vi "Multichannel Recording0.9B.vi"() -> ()   [LabVIEW 2014]
uses:
  Enum State Typedef.ctl
  Consumer Data_ Consumer Event Com.ctl
  Data Producer States.ctl
  <vilib>/_DAQmxBase/Internals/DAQmxBase Read (Analog 2D DBL NChan NSamp).vi
  <vilib>/_DAQmxBase/Internals/DAQmxBase Create Channel (AI-Voltage-Basic).vi
  <vilib>/_DAQmxBase/Internals/DAQmxBase Timing (Sample Clock).vi
panel:
  out "Recording Progress (% )":dbl(slide) scale=0.0..1.0
  in  "Display Size":T1(ring)
  out "Total Iterations Needed":dbl
  out "Read Data":i32
  out "Data Producer State":T2=enum."Default"
  out "Data Consumer State":T3=enum."Default"
  in  "Open Button":bool
  in  "Tab Control":T4(tab)
  in  "Amplifier Channel 0":T5 {"Amplifier Model" items=["Select a Model", "AM 1700", "BMA 200"]}
  out "Channel 0 Chart":waveform(dbl)(graph)
  in  "User Data Channel 0":T6
  in  "Use Channel 0":bool caption="In Use?"
  out "Channel 1 Chart":waveform(dbl)(graph)
  in  "User Data Channel 1":T6
  in  "Amplifier Channel 1":T5 {"Amplifier Model" items=["Select a Model", "AM 1700", "BMA 200"]}
  in  "Use Channel 1":bool caption="In Use?"
  out "Channel 2 Chart":waveform(dbl)(graph)
  in  "User Data Channel 2":T6
  in  "Amplifier Channel 2":T5 {"Amplifier Model" items=["Select a Model", "AM 1700", "BMA 200"]}
  in  "Use Channel 2":bool caption="In Use?"
  out "Channel 3 Chart":waveform(dbl)(graph)
  in  "User Data Channel 3":T6
  in  "Amplifier Channel 3":T5 {"Amplifier Model" items=["Select a Model", "AM 1700", "BMA 200"]}
  in  "Use Channel 3":bool caption="In Use?"
  out "Overview Chart":waveform(dbl)[](graph)
  in  "Stop Preview":bool
  in  "OK Button":bool
  out "Event State":T7
  in  "Clear Display":bool
  in  "Preview Button":bool
  out "Iterations Recorded":i32
  in  "Recording Time (s)":dbl
  in  "Sample Rate":i64=1000
  in  "Stop Button":bool
  out "Start Time hr/min":string
  out "Date mm/dd/yy":string
  in  "Exit Button":bool
  in  "Record Button":bool
  # "MSU EFISH Lab Multi-Channel Electronic Pulse Recorder v0.9A (Beta 2)"
  # "Setup"
  # "Must set sample rate before you press start"
  # "Preview"
  # "Recording"
  # "Blue for On\nOrange for Off"
  # "DC"
  # "AC"
  # "Blue for AC and Orange for DC"
  # "Blue for On\nOrange for Off"
  # "DC"
  # "AC"
  # "Blue for AC and Orange for DC"
  # "Blue for On\nOrange for Off"
  # "DC"
  # "AC"
  # "Blue for AC and Orange for DC"
  # "Blue for On\nOrange for Off"
  # "DC"
  # "AC"
  # "Blue for AC and Orange for DC"
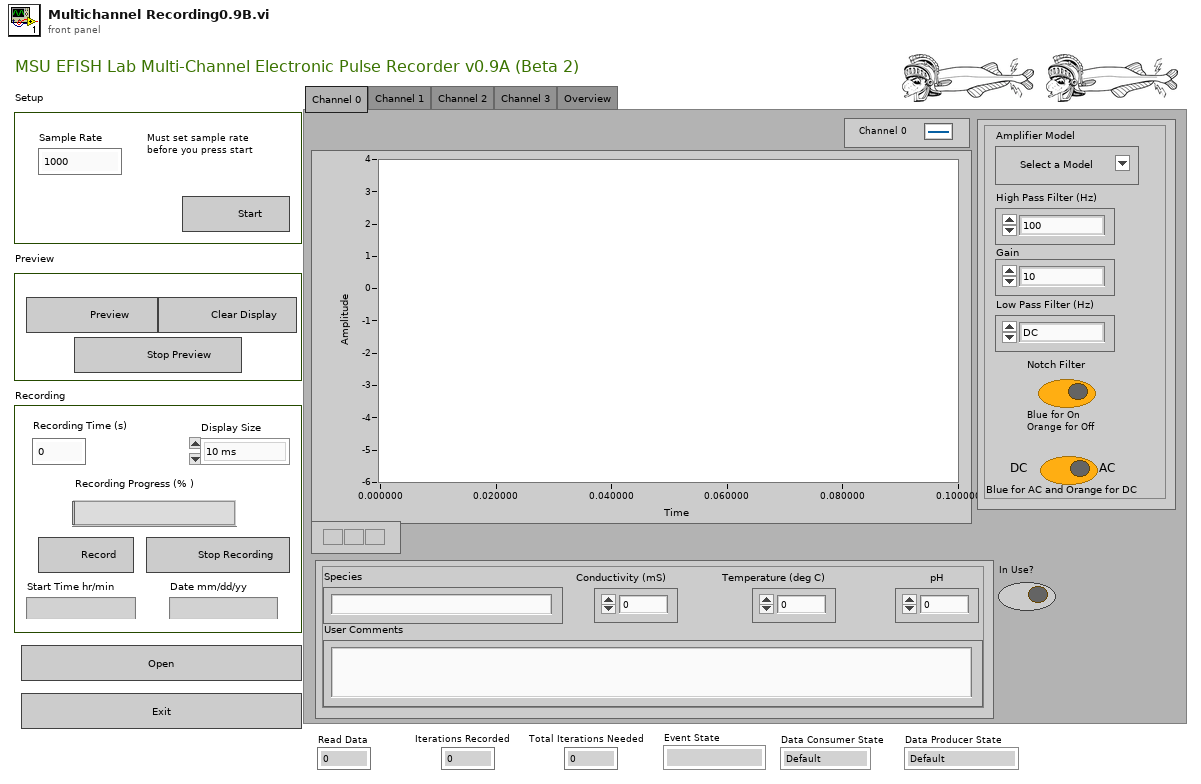
[diagram p1: front panel]
types:
  T1 = enum16{"10 ms", "100 ms", "1 Second", "10 sec", "30 sec"}
  T2 = typedef "Data Producer States.ctl" = enum16{"Read Data", "Set Sample Clock", "Default", "Exit", "Preview"}
  T3 = typedef "Consumer Data_ Consumer Event Com.ctl" = enum16{"Recording", "Create File", "Clear Memory", "Default", "End File", "Exit", "Set Sample Clock", "Preview"}
  T4 = enum32{"Channel 0", "Channel 1", "Channel 2", "Channel 3", "Overview"}
  T5 = cluster{"Low Pass Filter (Hz)":enum16{"DC", "0.1", "1", "3", "10", "30", "100", "300"}, "Gain ":enum16{"10", "20", "50", "100", "200", "500", "1000", "2k", "5k", "10k", "20k", "50k"}, "High Pass Filter (Hz)":enum16{"100", "500", "1000", "3000", "5000", "10,000", "20,000", "30,000", "50,000"}, "Notch Filter":bool, "Amplifier Model":u16, "AC/DC Switch":bool}
  T6 = cluster{"pH":dbl, "Conductivity (mS)":dbl, "Temperature (deg C)":dbl, "User Comments":string, "Species":string}
  T7 = typedef "Enum State Typedef.ctl" = enum16{"", "Open FIle", "Beginning State", "Set the Sample Clock", "Prepreview Handling", "Clear Display", "Preview Data", "Stop", "Exit", "Record", "Create File"}
  T8 = enum8{"Enabled", "Disabled", "Disabled and Grayed Out"}
  T9 = enum16{"Recording", "Create File", "Clear Memory", "Default"}
  T10 = cluster{"Refnum out":refnum<k34>, "Refnum out":refnum<k34>, "Refnum out":refnum<k34>, "Refnum out":refnum<k34>}
  T11 = cluster{"Use Channel 0":bool, "Use Channel 1":bool, "Use Channel 2":bool, "Use Channel 3":bool}
  T12 = cluster{"tdms file out":refnum<k34>, "tdms file out":refnum<k34>, "tdms file out":refnum<k34>, "tdms file out":refnum<k34>}
  T13 = cluster{"Waveform":waveform(dbl), "Waveform":waveform(dbl), "Waveform":waveform(dbl), "Waveform":waveform(dbl), waveform(dbl)[]}
  T14 = cluster{"Channel 0 Chart":refnum<vi>, "Channel 1 Chart":refnum<vi>, "Channel 2 Chart":refnum<vi>, "Channel 3 Chart":refnum<vi>, "Overview Chart":refnum<vi>}
  T15 = enum16{"Read Data", "Set Sample Clock", "Default", "Exit"}
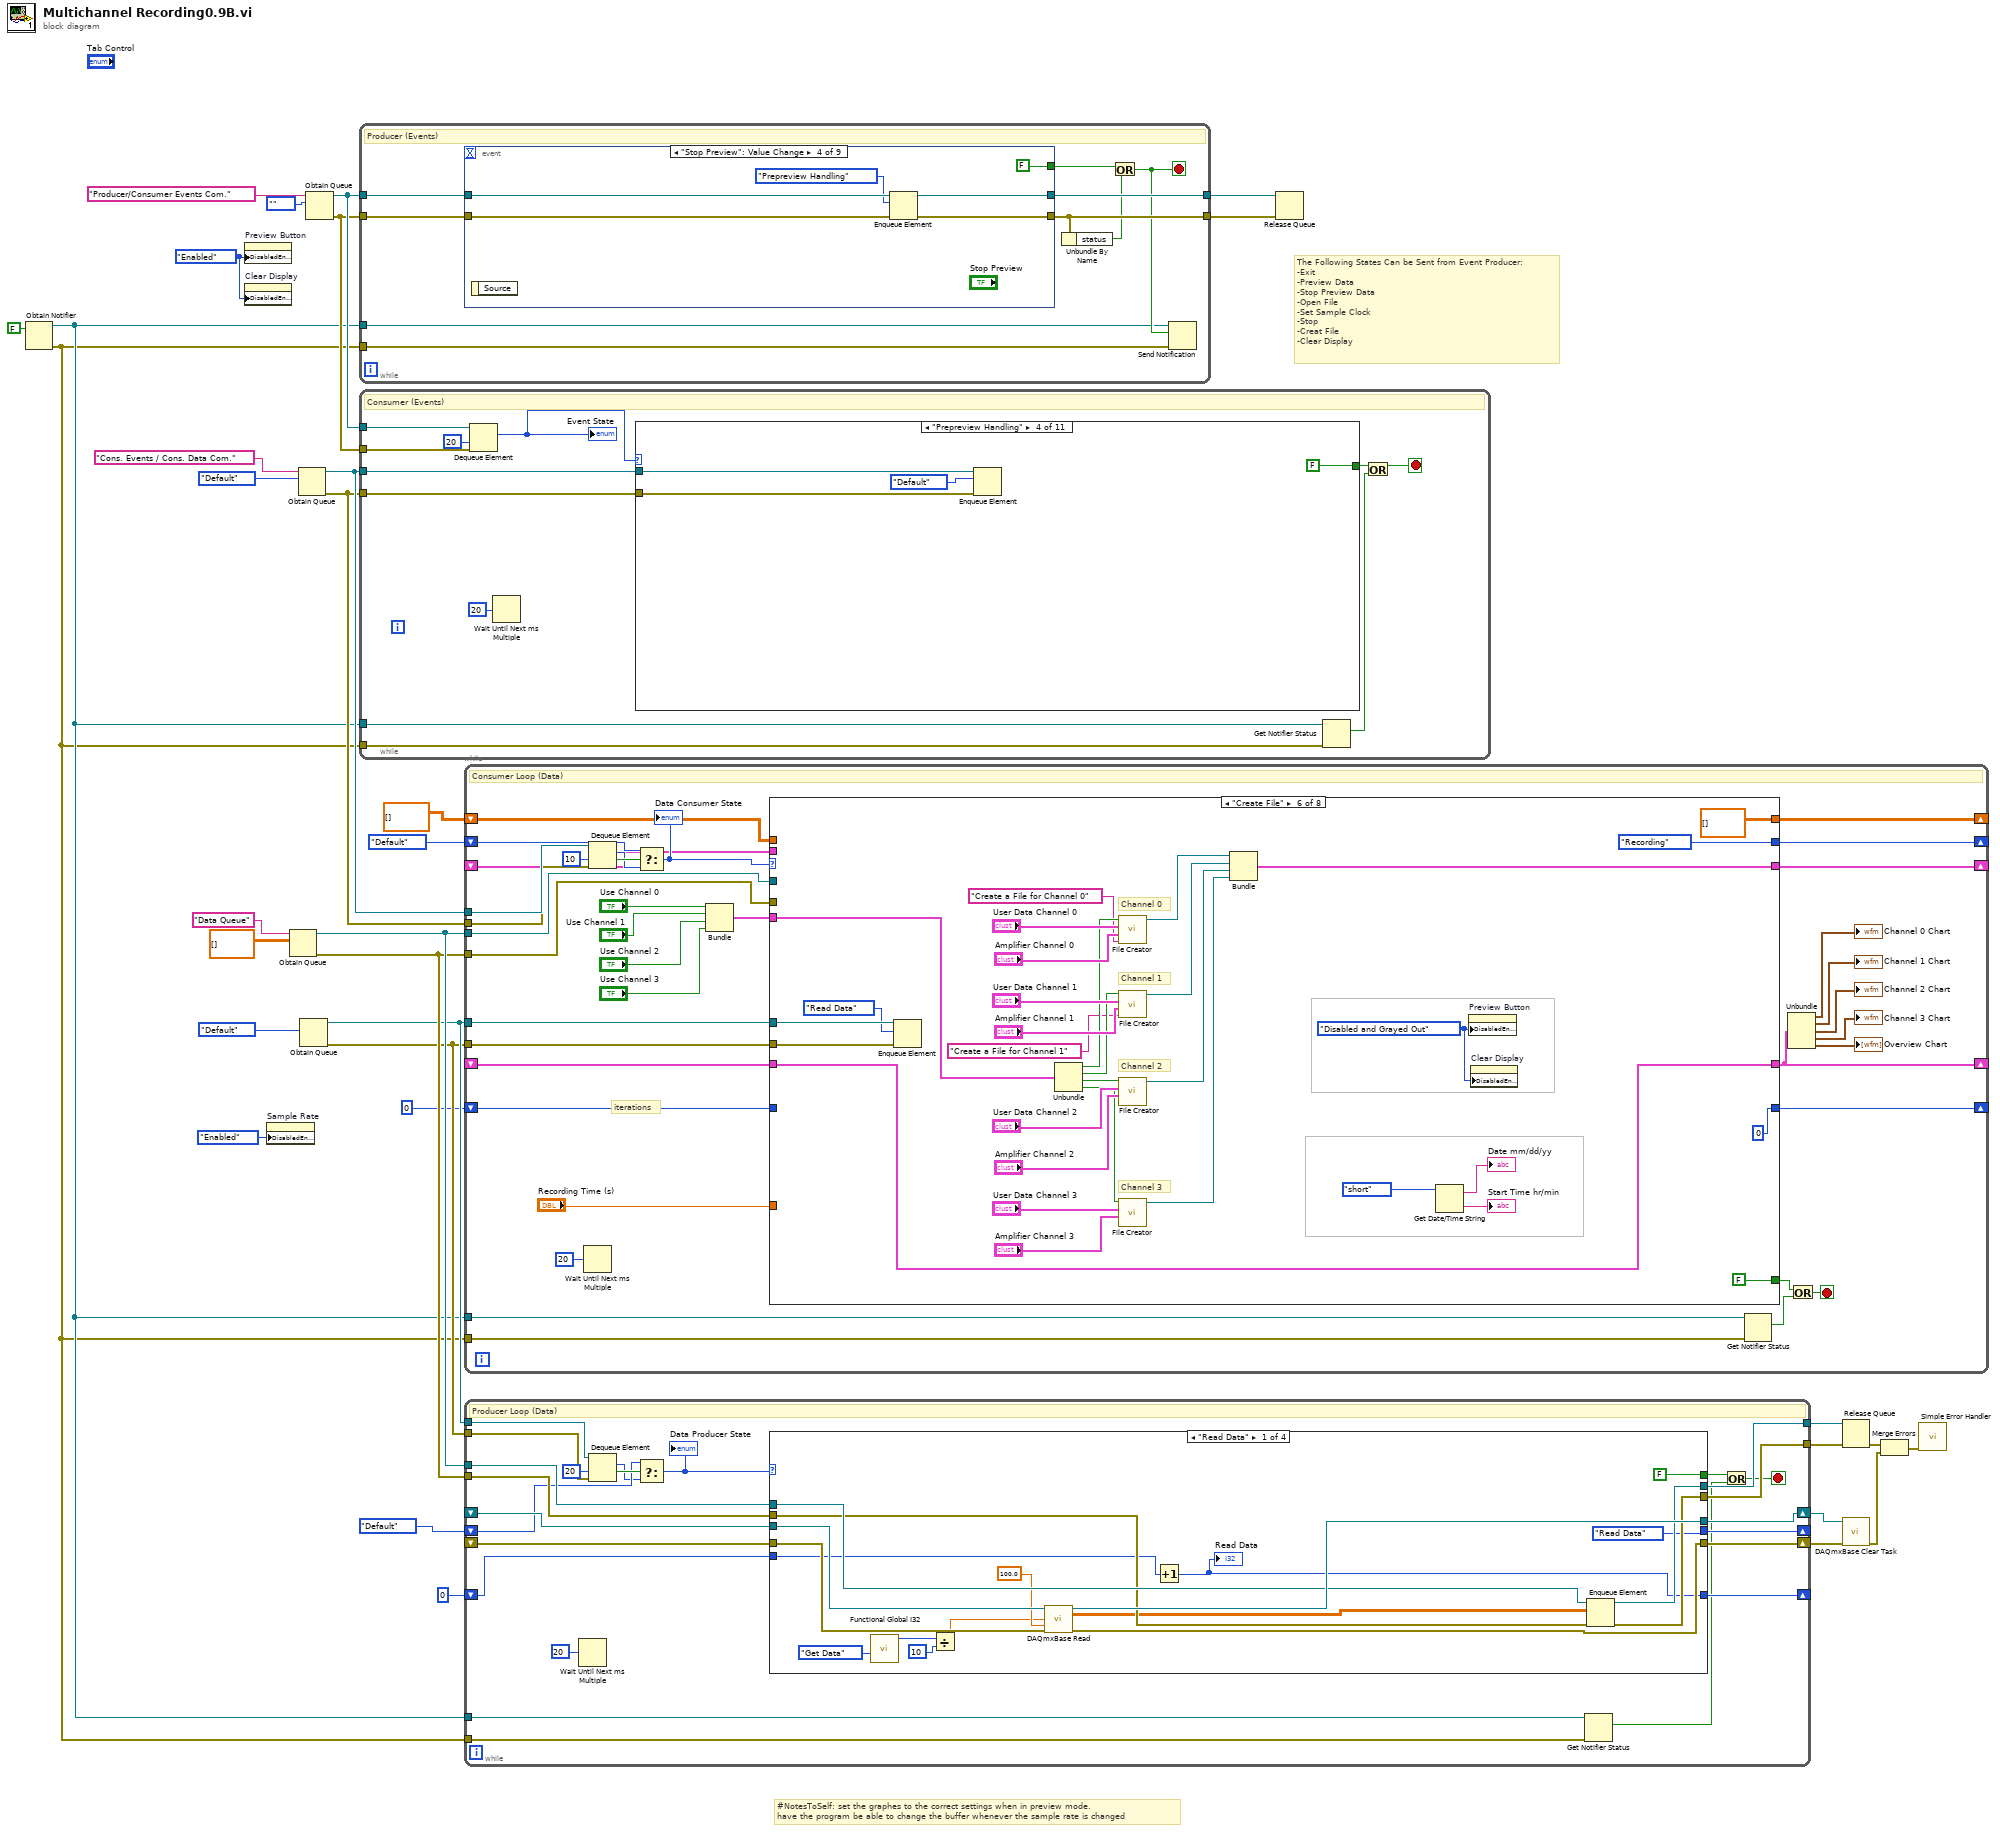
[diagram p0: block diagram]
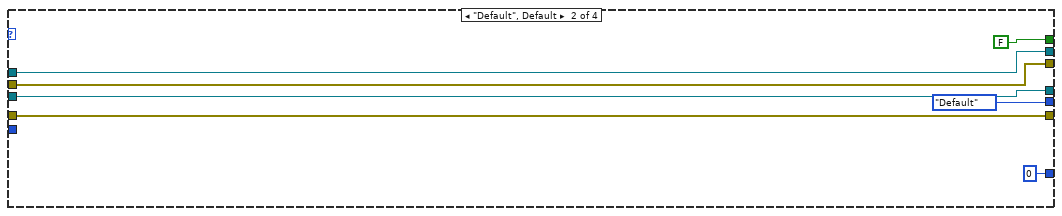
[diagram p2: hidden frame]
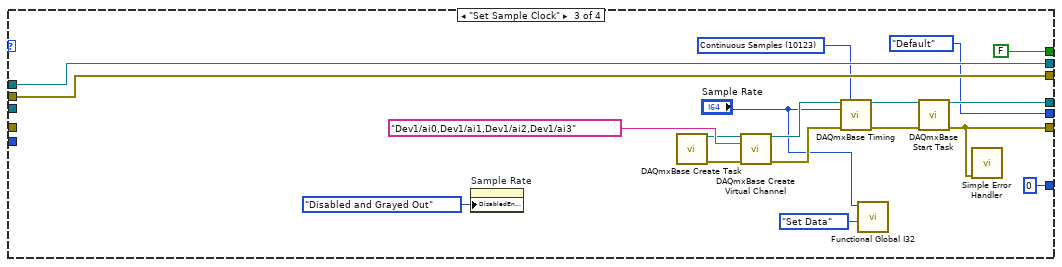
[diagram p3: hidden frame]
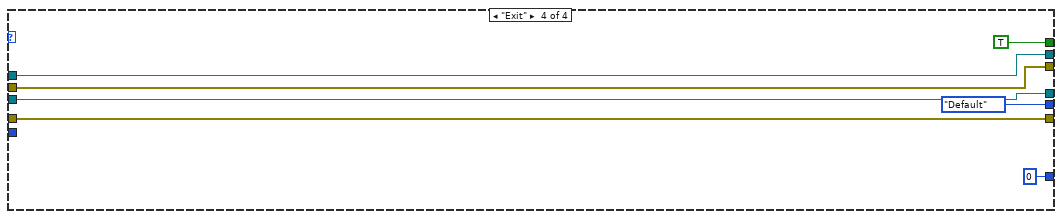
[diagram p4: hidden frame]
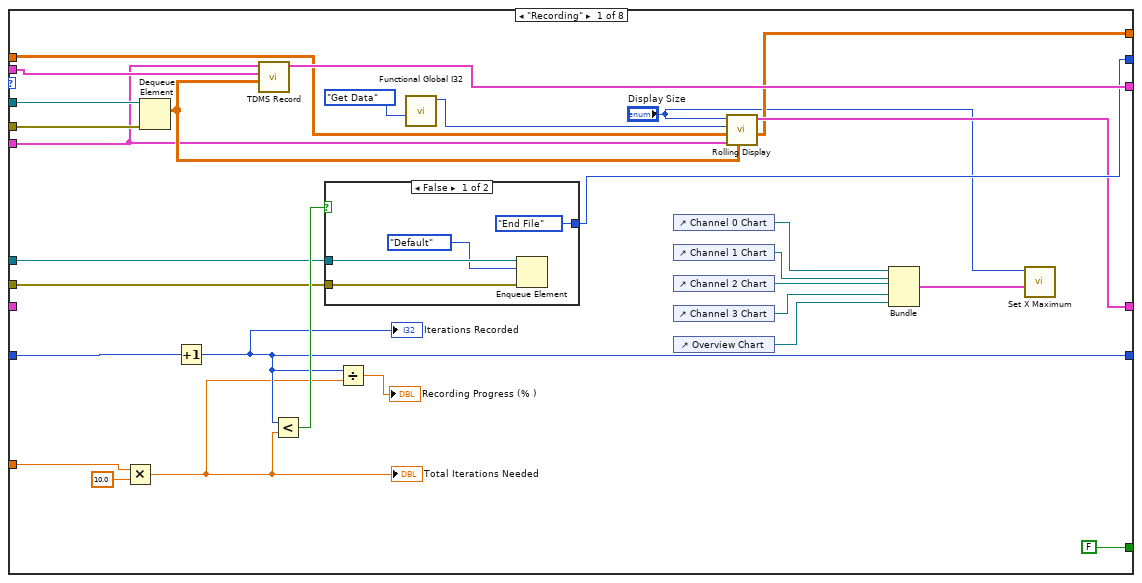
[diagram p5: hidden frame]
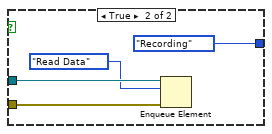
[diagram p6: hidden frame]
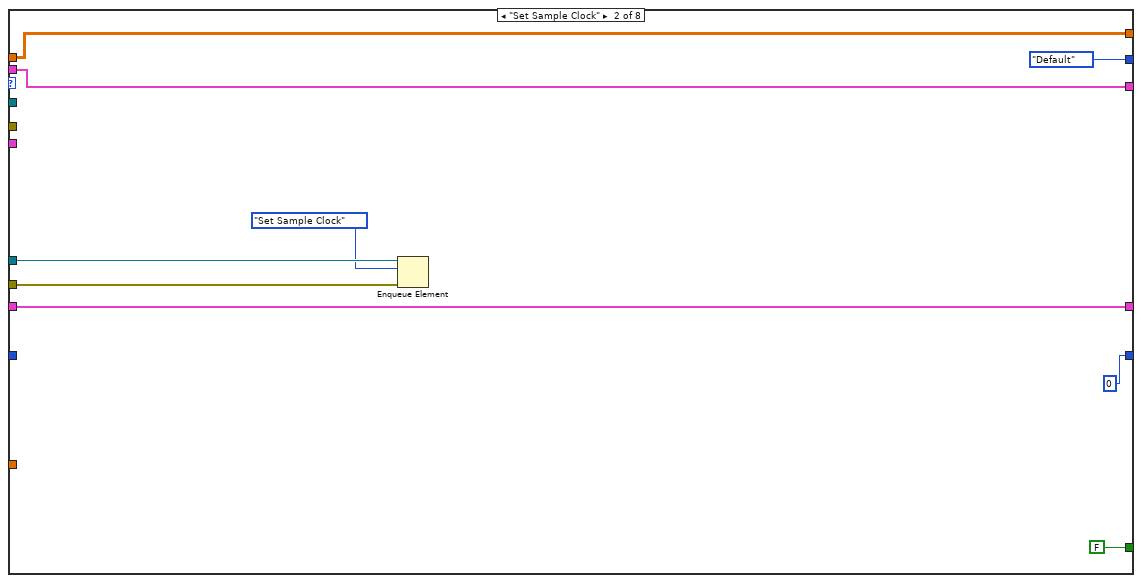
[diagram p7: hidden frame]
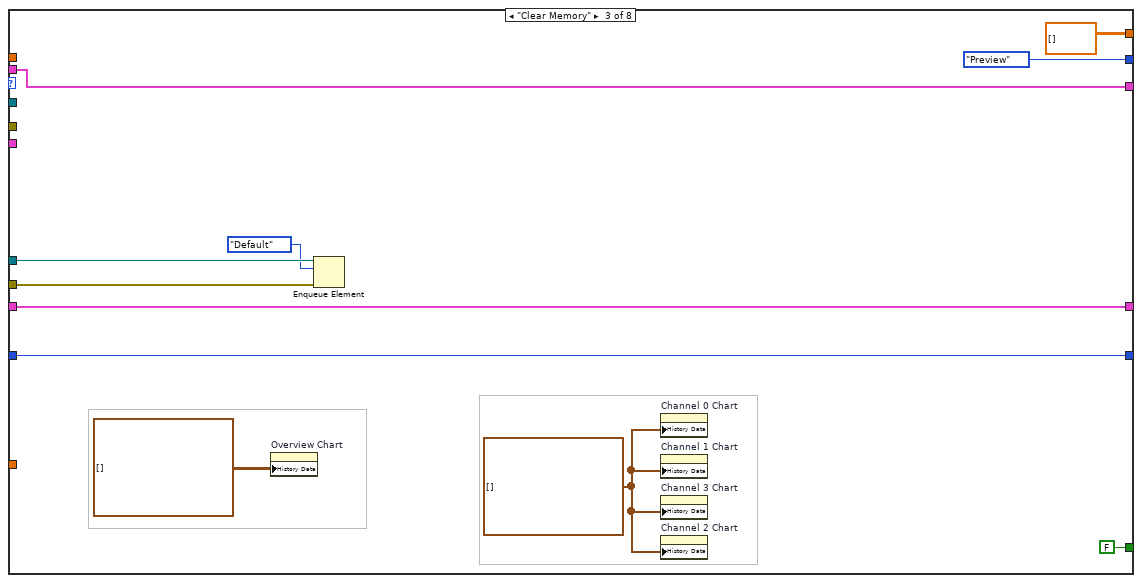
[diagram p8: hidden frame]
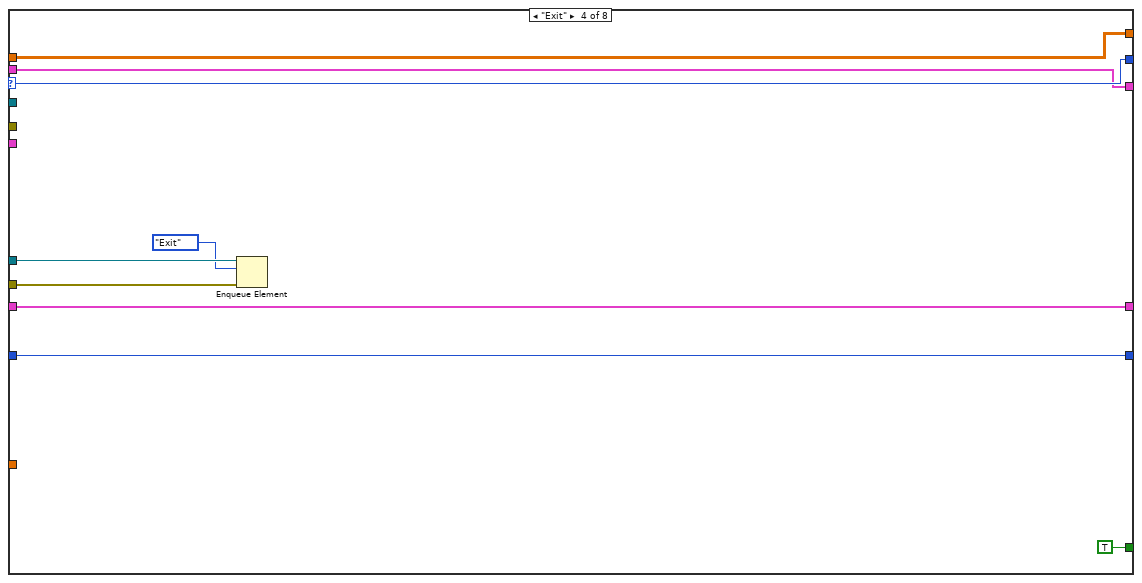
[diagram p9: hidden frame]
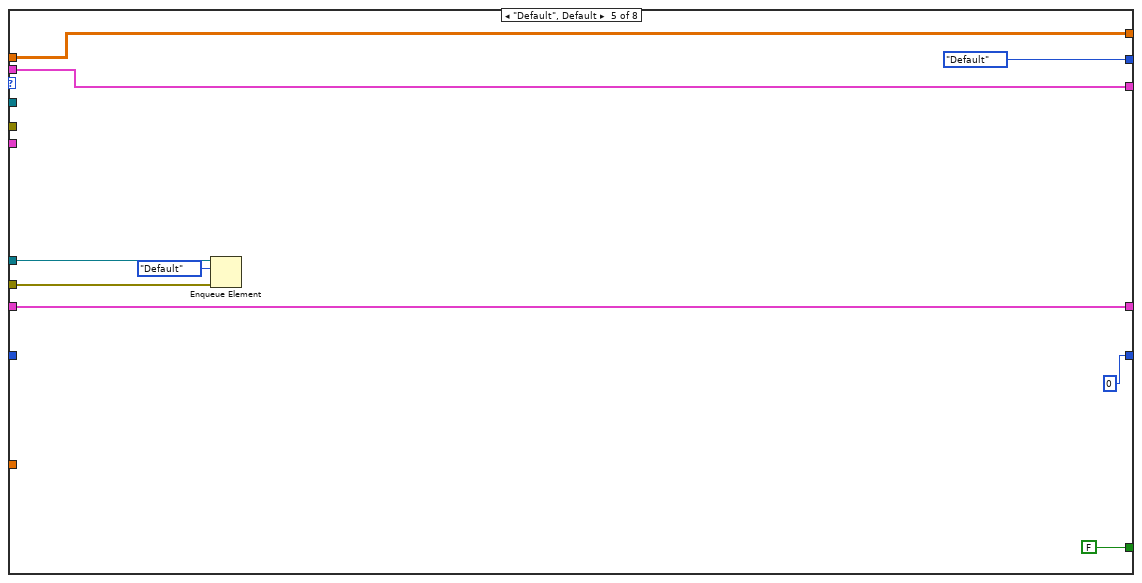
[diagram p10: hidden frame]
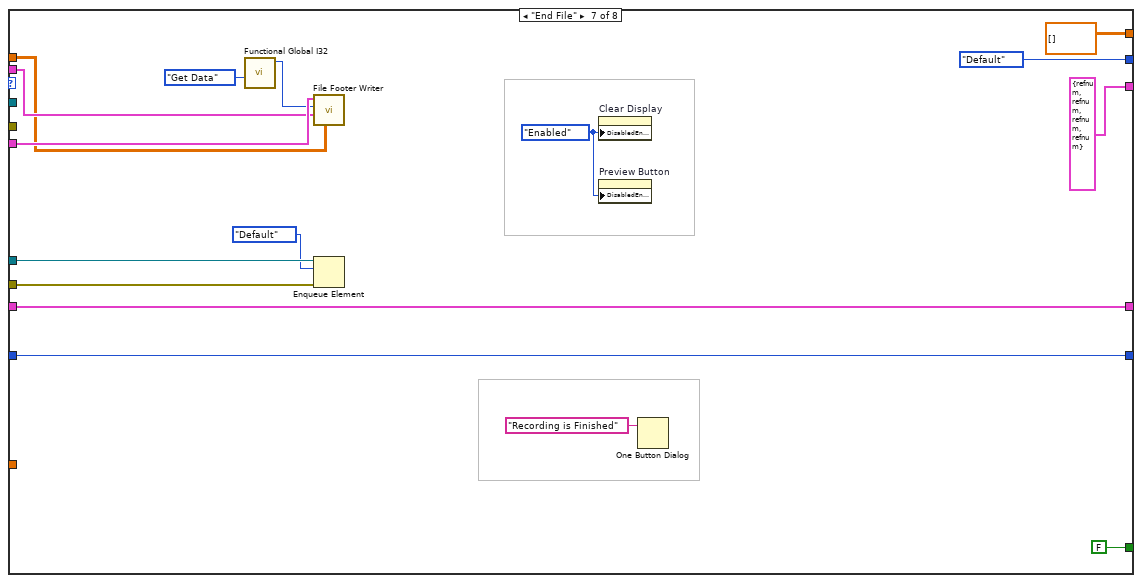
[diagram p11: hidden frame]
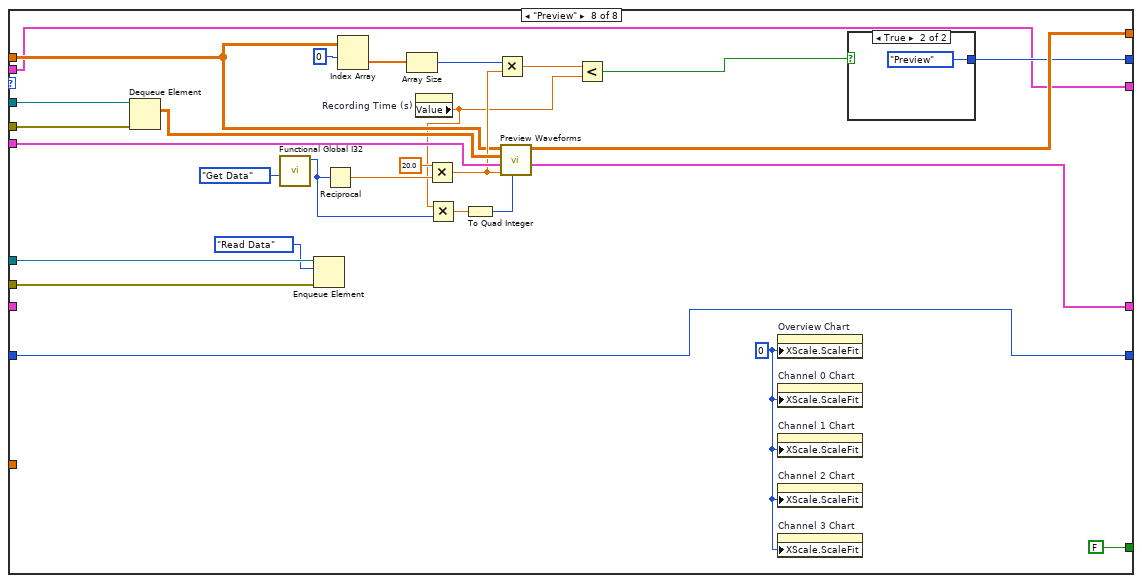
[diagram p12: hidden frame]
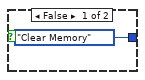
[diagram p13: hidden frame]
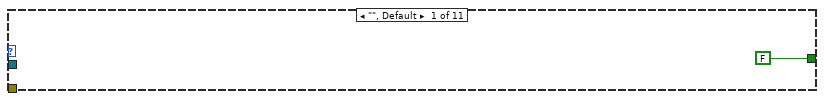
[diagram p14: hidden frame]
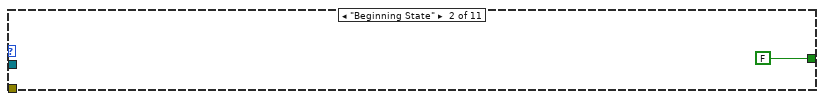
[diagram p15: hidden frame]
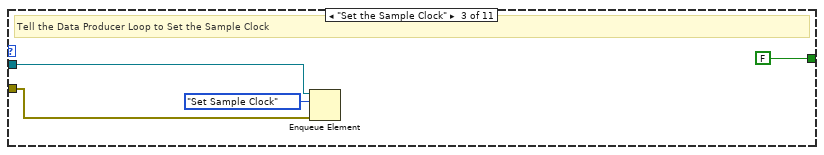
[diagram p16: hidden frame]
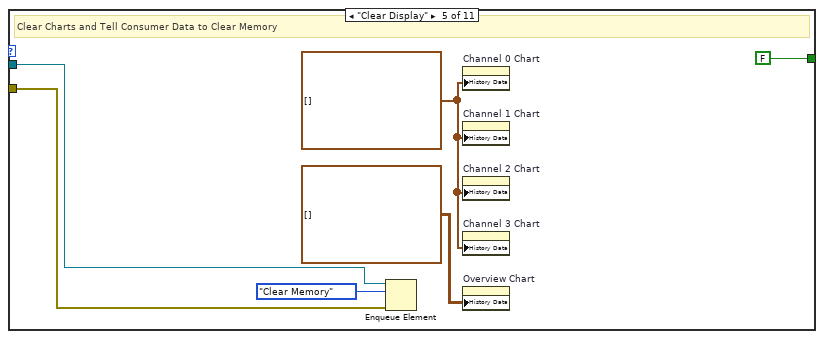
[diagram p17: hidden frame]
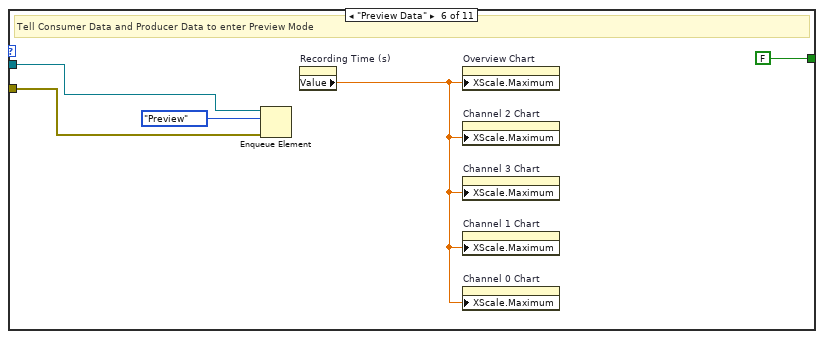
[diagram p18: hidden frame]
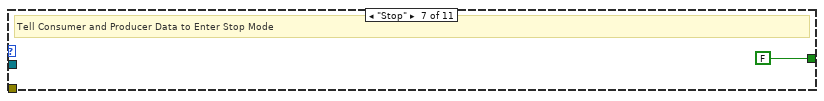
[diagram p19: hidden frame]
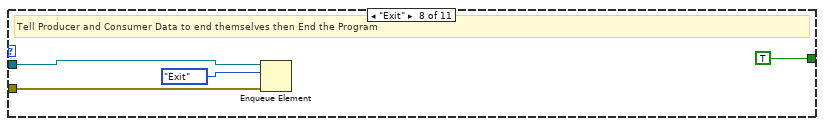
[diagram p20: hidden frame]
diagram:
  w1 = T8."Enabled" ("Disabled")
  # "#NotesToSelf: set the graphes to the correct settings when in preview mode.\nhave the program be able to change the buffer whenever the sample rate is changed"
  # "The Following States Can be Sent from Event Producer:\n-Exit\n-Preview Data\n-Stop Preview Data\n-Open File\n-Set Sample Clock\n-Stop\n-Creat File\n-Clear Display"
  n1 = Obtain Notifier(notification data type=FALSE) -> (notifier out=w3:refnum<notifier>, error out=w2:errorcluster)  [unwired: 3 in, 1 out]
  n2 = property on="Preview Button" class="Bool (strict)"("DisabledEnum"=w1) -> ()  [unwired: 2 in, 2 out]
  n3 = property on="Clear Display" class="Bool"("DisabledEnum"=w1) -> ()  [unwired: 2 in, 2 out]
  n4 = property on="Sample Rate" class="DigNum (strict)"("DisabledEnum"=T8."Enabled" ("Disabled")) -> ()  [unwired: 2 in, 2 out]
  n5 = Obtain Queue(name (unnamed)="Data Queue", element data type=dbl[][] []) -> (queue out=w29:refnum<queue>, error out=w28:errorcluster)  [unwired: 3 in, 1 out]
  n6 = Obtain Queue(name (unnamed)="Cons. Events / Cons. Data Com.", element data type=Consumer_Data__Consumer_Event_Com."Default") -> (queue out=w21:refnum<queue>, error out=w20:errorcluster)  [unwired: 3 in, 1 out]
  n7 = Obtain Queue(element data type=Data_Producer_States."Default") -> (queue out=w10:refnum<queue>, error out=w9:errorcluster)  [unwired: 4 in, 1 out]
  n8 = Obtain Queue(name (unnamed)="Producer/Consumer Events Com.", element data type=Enum_State_Typedef."" ("State")) -> (queue out=w33:refnum<queue>, error out=w32:errorcluster)  [unwired: 3 in, 1 out]
  n9 = while {
    tunnel: w33 -> [w43]
    tunnel: w32 -> [w42]
    tunnel: [w41] -> w27
    tunnel: [w40] -> w26
    tunnel: w3 -> [w36]
    tunnel: w2 -> [w35]
    stop <- w37 stop-if-true
    # "Producer (Events)"
    n10 = event shown="[3] \"Stop Preview\": Value Change" {
      selector: _ -> [_ _ _ _ _ _ _ _ _]
      dyn-events: _ -> [_ _ _ _ _ _ _ _ _]
      timeout: _ -> [_ _ _ _ _ _ _ _ _]
      tunnel: [FALSE ("Exit Button") "Exit Button" FALSE ("Exit Button") FALSE ("Exit Button") FALSE ("Exit Button") FALSE ("Exit Button") FALSE ("Exit Button") FALSE ("Exit Button") FALSE ("Exit Button")] -> w39
      tunnel: w43 -> [w45 w51 w58 w64 w70 w76 w82 w88 w94]
      tunnel: w42 -> [w44 w50 w57 w63 w69 w75 w81 w87 w93]
      tunnel: [w45 w48 w54 w60 w66 w72 w78 w84 w90] -> w41
      tunnel: [w44 w47 w53 w59 w65 w71 w77 w83 w89] -> w40
      event Timeout {
        n11 = event-data() -> ()  [unwired: 1 in, 1 out]
      }
      event "Exit Button": Value Change {
        n12 = event-data() -> ()  [unwired: 1 in, 1 out]
        n13 = Enqueue Element(queue=w51, element=Enum_State_Typedef."Exit", error in (no error)=w50) -> (queue out=w48:refnum<queue>, error out=w47:errorcluster)  [unwired: 1 in, 1 out]
      }
      event "Preview Button": Value Change {
        n14 = event-data() -> ()  [unwired: 1 in, 1 out]
        n15 = Enqueue Element(queue=w58, element=Enum_State_Typedef."Preview Data", error in (no error)=w57) -> (queue out=w54:refnum<queue>, error out=w53:errorcluster)  [unwired: 1 in, 1 out]
      }
      event "Stop Preview": Value Change {
        n16 = event-data() -> ()  [unwired: 1 in, 1 out]
        n17 = Enqueue Element(queue=w64, element=Enum_State_Typedef."Prepreview Handling", error in (no error)=w63) -> (queue out=w60:refnum<queue>, error out=w59:errorcluster)  [unwired: 1 in, 1 out]
      }
      event "Open Button": Value Change {
        n18 = event-data() -> ()  [unwired: 1 in, 1 out]
        n19 = Enqueue Element(queue=w70, element=Enum_State_Typedef."Open FIle", error in (no error)=w69) -> (queue out=w66:refnum<queue>, error out=w65:errorcluster)  [unwired: 1 in, 1 out]
      }
      event "OK Button": Value Change {
        n20 = event-data() -> ()  [unwired: 1 in, 1 out]
        n21 = Enqueue Element(queue=w76, element=Enum_State_Typedef."Set the Sample Clock", error in (no error)=w75) -> (queue out=w72:refnum<queue>, error out=w71:errorcluster)  [unwired: 1 in, 1 out]
      }
      event "Stop Button": Value Change {
        n22 = event-data() -> ()  [unwired: 1 in, 1 out]
        n23 = Enqueue Element(queue=w82, element=Enum_State_Typedef."Stop", error in (no error)=w81) -> (queue out=w78:refnum<queue>, error out=w77:errorcluster)  [unwired: 1 in, 1 out]
      }
      event "Record Button": Value Change {
        n24 = event-data() -> ()  [unwired: 1 in, 1 out]
        n25 = Enqueue Element(queue=w88, element=Enum_State_Typedef."Create File", error in (no error)=w87) -> (queue out=w84:refnum<queue>, error out=w83:errorcluster)  [unwired: 1 in, 1 out]
      }
      event "Clear Display": Value Change {
        n26 = event-data() -> ()  [unwired: 1 in, 1 out]
        n27 = Enqueue Element(queue=w94, element=Enum_State_Typedef."Clear Display", error in (no error)=w93) -> (queue out=w90:refnum<queue>, error out=w89:errorcluster)  [unwired: 1 in, 1 out]
      }
    }
    n28 = Unbundle By Name(w40) -> ("status"=w38:bool)
    n29 = Or(x=w39, y=w38) -> (x .or. y?=w37:bool)
    n30 = Send Notification(notification=w37, notifier=w36, error in (no error)=w35) -> ()  [unwired: 2 out]
  }
  n31 = while {
    tunnel: w33 -> [w106]
    tunnel: w32 -> [w105]
    tunnel: w21 -> [w104]
    tunnel: w20 -> [w103]
    tunnel: w3 -> [w98]
    tunnel: w2 -> [w97]
    stop <- w96 stop-if-true
    # "Consumer (Events)"
    n32 = Dequeue Element(queue=w106, timeout in ms (-1)=20, error in (no error)=w105) -> (element=w101:T7)  [unwired: 3 out]
    "Event State" <- w101
    n33 = Wait Until Next ms Multiple(millisecond multiple=u32 20) -> ()  [unwired: 1 out]
    n34 = case shown="\"Prepreview Handling\"" w101 {
      tunnel: w104 -> [_ _ w111 w115 w119 w125 _ w132 _ w137 _]
      tunnel: w103 -> [_ _ w110 w114 w118 w124 _ w131 _ w136 _]
      tunnel: [FALSE FALSE FALSE FALSE FALSE FALSE FALSE TRUE FALSE FALSE FALSE] -> w102
      frame "", Default {
      }
      frame "Beginning State" {
      }
      frame "Set the Sample Clock" {
        # "Tell the Data Producer Loop to Set the Sample Clock"
        n35 = Enqueue Element(queue=w111, element=Consumer_Data__Consumer_Event_Com."Set Sample Clock", error in (no error)=w110) -> ()  [unwired: 1 in, 3 out]
      }
      frame "Prepreview Handling" {
        n36 = Enqueue Element(queue=w115, element=Consumer_Data__Consumer_Event_Com."Default", error in (no error)=w114) -> ()  [unwired: 1 in, 3 out]
      }
      frame "Clear Display" {
        w121 = waveform(dbl)[] [] ("History Data")
        # "Clear Charts and Tell Consumer Data to Clear Memory"
        n37 = Enqueue Element(queue=w119, element=Consumer_Data__Consumer_Event_Com."Clear Memory", error in (no error)=w118) -> ()  [unwired: 1 in, 3 out]
        n38 = property on="Channel 0 Chart" class="WFChart (strict)"("History Data"=w121) -> ()  [unwired: 2 in, 2 out]
        n39 = property on="Channel 1 Chart" class="WFChart (strict)"("History Data"=w121) -> ()  [unwired: 2 in, 2 out]
        n40 = property on="Channel 2 Chart" class="WFChart (strict)"("History Data"=w121) -> ()  [unwired: 2 in, 2 out]
        n41 = property on="Channel 3 Chart" class="WFChart (strict)"("History Data"=w121) -> ()  [unwired: 2 in, 2 out]
        n42 = property on="Overview Chart" class="WFChart (strict)"("History Data"=waveform(dbl)[][] []) -> ()  [unwired: 2 in, 2 out]
      }
      frame "Preview Data" {
        # "Tell Consumer Data and Producer Data to enter Preview Mode"
        n43 = Enqueue Element(queue=w125, element=Consumer_Data__Consumer_Event_Com."Preview", error in (no error)=w124) -> ()  [unwired: 1 in, 3 out]
        n44 = property on="Recording Time (s)" class="DigNum (strict)"() -> ("Value"=w126:dbl)  [unwired: 2 in, 2 out]
        n45 = property on="Overview Chart" class="WFChart (strict)"("XScale.Maximum"=w126) -> ()  [unwired: 2 in, 2 out]
        n46 = property on="Channel 2 Chart" class="WFChart (strict)"("XScale.Maximum"=w126) -> ()  [unwired: 2 in, 2 out]
        n47 = property on="Channel 3 Chart" class="WFChart (strict)"("XScale.Maximum"=w126) -> ()  [unwired: 2 in, 2 out]
        n48 = property on="Channel 1 Chart" class="WFChart (strict)"("XScale.Maximum"=w126) -> ()  [unwired: 2 in, 2 out]
        n49 = property on="Channel 0 Chart" class="WFChart (strict)"("XScale.Maximum"=w126) -> ()  [unwired: 2 in, 2 out]
      }
      frame "Stop" {
        # "Tell Consumer and Producer Data to Enter Stop Mode"
      }
      frame "Exit" {
        # "Tell Producer and Consumer Data to end themselves then End the Program"
        n50 = Enqueue Element(queue=w132, element=Consumer_Data__Consumer_Event_Com."Exit", error in (no error)=w131) -> ()  [unwired: 1 in, 3 out]
      }
      frame "Record" {
        # "(I dont think that this case will exist)"
      }
      frame "Create File" {
        w134 = u8 0 ("X Scale.Scale Fit")
        # "Let Consumer Data Create File"
        n51 = Enqueue Element(queue=w137, element=Consumer_Data__Consumer_Event_Com."Create File", error in (no error)=w136) -> ()  [unwired: 1 in, 3 out]
        n52 = property on="Overview Chart" class="WFChart (strict)"("XScale.ScaleFit"=w134) -> ()  [unwired: 2 in, 2 out]
        n53 = property on="Channel 3 Chart" class="WFChart (strict)"("XScale.ScaleFit"=w134) -> ()  [unwired: 2 in, 2 out]
        n54 = property on="Channel 2 Chart" class="WFChart (strict)"("XScale.ScaleFit"=w134) -> ()  [unwired: 2 in, 2 out]
        n55 = property on="Channel 1 Chart" class="WFChart (strict)"("XScale.ScaleFit"=w134) -> ()  [unwired: 2 in, 2 out]
        n56 = property on="Channel 0 Chart" class="WFChart (strict)"("XScale.ScaleFit"=w134) -> ()  [unwired: 2 in, 2 out]
      }
      frame "Open FIle" {
        # "Tell the Data Consumer to Create the File"
        n57 = call "File Dialog"() -> ("selected path"=w139:path)  [unwired: 12 in, 3 out]
        n58 = call <vilib>:"TDMS - File Viewer.vi"("file path"=w139) -> ()  [unwired: 5 in, 2 out]
      }
    }
    n59 = Get Notifier Status(notifier=w98, error in (no error)=w97) -> (current notification=w95:bool)  [unwired: 4 out]
    n60 = Or(x=w102, y=w95) -> (x .or. y?=w96:bool)
  }
  n61 = while {
    tunnel: w29 -> [w170]
    tunnel: w28 -> [w169]
    tunnel: w21 -> [w177]
    tunnel: w20 -> [w176]
    shift-right: [w171] -> _
    shift-left: Consumer_Data__Consumer_Event_Com."Default" -> [w172]
    shift-right: [w165] -> _
    shift-left: dbl[][] [] -> [w168]
    shift-right: [w164] -> _
    shift-left: _ -> [w163]
    tunnel: w10 -> [w161]
    tunnel: w9 -> [w160]
    shift-right: [w156] -> _
    shift-left: 0 -> [w158]
    tunnel: w3 -> [w150]
    tunnel: w2 -> [w149]
    shift-right: [w142] -> _
    shift-left: _ -> [w141]
    stop <- w152 stop-if-true
    # "iterations"
    # "Consumer Loop (Data)"
    n62 = Wait Until Next ms Multiple(millisecond multiple=u32 20) -> ()  [unwired: 1 out]
    n63 = Dequeue Element(queue=w177, timeout in ms (-1)=10, error in (no error)=w176) -> (element=w174:T3, timed out?=w175:bool)  [unwired: 2 out]
    n64 = Select(t=w172, s=w175, f=w174) -> (s? t:f=w173:T3)
    "Data Consumer State" <- w173
    n65 = Bundle("Use Channel 0"="Use Channel 0", "Use Channel 1"="Use Channel 1", "Use Channel 2"="Use Channel 2", "Use Channel 3"="Use Channel 3") -> (w166:T11)  [unwired: 1 in]
    n66 = case shown="\"Create File\"" w173 {
      selector: w173 -> [_ _ _ w241 _ _ _ _]
      tunnel: [w198 Consumer_Data__Consumer_Event_Com."Default" Consumer_Data__Consumer_Event_Com."Preview" w241 T9."Default" Consumer_Data__Consumer_Event_Com."Recording" Consumer_Data__Consumer_Event_Com."Default" w314] -> w171
      tunnel: w170 -> [w205 _ _ _ _ _ _ w328]
      tunnel: w169 -> [w204 _ _ _ _ _ _ w327]
      tunnel: [FALSE FALSE FALSE TRUE FALSE FALSE FALSE FALSE] -> w151
      tunnel: w168 -> [w191 w220 _ w242 w250 _ w298 w320]
      tunnel: w166 -> [w190 _ _ _ _ w278 w300 w325]
      tunnel: [w188 w220 dbl[][] [] ("Output Decimated Data") w242 w250 dbl[][] [] ("Output Decimated Data") dbl[][] [] ("Output Data") w322] -> w165
      tunnel: [w203 w219 w231 w240 w249 w261 T10 {"Refnum out"=refnum, "Refnum out"=refnum, "Refnum out"=refnum, "Refnum out"=refnum} ("Output TDMS File Cluster") w301] -> w164
      tunnel: w163 -> [w195 w219 w231 w240 w249 _ w299 w301]
      tunnel: w161 -> [w197 w223 w228 w239 w247 w260 w293 w312]
      tunnel: w160 -> [w196 w222 w227 w238 w246 w259 w292 w311]
      tunnel: w158 -> [w202 _ w225 w236 _ _ w290 w309]
      tunnel: "Recording Time (s)" -> [w201 _ _ _ _ _ _ _]
      tunnel: [w180 0 w225 w236 0 0 w290 w309] -> w156
      tunnel: [w189 w215 w224 w235 w244 w254 w288 w306] -> w142
      tunnel: w141 -> [_ w215 w224 w235 w244 w254 w288 _]
      frame "Recording" {
        n67 = Multiply(x=w201, y=10.0) -> (x*y=w179:dbl)
        "Total Iterations Needed" <- w179
        n68 = Dequeue Element(queue=w205, error in (no error)=w204) -> (element=w192:dbl[][])  [unwired: 1 in, 3 out]
        n69 = Increment(x=w202) -> (x+1=w180:i32)
        "Iterations Recorded" <- w180
        n70 = call "TDMS Record.vi"("Data"=w192, "Input TDMS File Cluster"=w195, "In Use Cluster"=w190) -> ("Output TDMS File Cluster"=w203:T12)  [unwired: 8 in]
        n71 = Less?(x=w180, y=w179) -> (x < y?=w199:bool)
        n72 = case shown="False" w199 {
          tunnel: [Consumer_Data__Consumer_Event_Com."End File" Consumer_Data__Consumer_Event_Com."Recording"] -> w198
          tunnel: w197 -> [w209 w213]
          tunnel: w196 -> [w208 w212]
          frame False {
            n73 = Enqueue Element(queue=w209, element=Data_Producer_States."Default", error in (no error)=w208) -> ()  [unwired: 1 in, 3 out]
          }
          frame True {
            n74 = Enqueue Element(queue=w213, element=Data_Producer_States."Read Data", error in (no error)=w212) -> ()  [unwired: 1 in, 3 out]
          }
        }
        n75 = Divide(x=w180, y=w179) -> (x/y=→"Recording Progress (% )":dbl)
        n76 = call "Functional Global I32.vi"("Enum"=enum16{"Set Data", "Get Data"}."Get Data") -> ("Integer"=w193:i32)  [unwired: 10 in]
        n77 = control-ref of="Channel 0 Chart"() -> (w187:refnum<vi>)
        n78 = control-ref of="Channel 1 Chart"() -> (w186:refnum<vi>)
        n79 = control-ref of="Channel 2 Chart"() -> (w185:refnum<vi>)
        n80 = control-ref of="Channel 3 Chart"() -> (w184:refnum<vi>)
        n81 = control-ref of="Overview Chart"() -> (w183:refnum<vi>)
        n82 = call "Rolling Display.vi"("Input Data"=w192, "Channels in Use"=w190, "Old Data"=w191, "Sample Rate"=w193, "Display Size"="Display Size") -> ("Output Array Values"=w188:dbl[][], "Output Waveform Cluster"=w189:T13)  [unwired: 5 in]
        n83 = Bundle("Channel 0 Chart"=w187, "Channel 1 Chart"=w186, "Channel 2 Chart"=w185, "Channel 3 Chart"=w184, "Overview Chart"=w183) -> (w182:T14)  [unwired: 1 in]
        n84 = call "Set X Maximum.vi"("Waveform Reference Cluster"=w182, "Display Size"="Display Size") -> ()  [unwired: 10 in]
      }
      frame "Set Sample Clock" {
        n85 = Enqueue Element(queue=w223, element=Data_Producer_States."Set Sample Clock", error in (no error)=w222) -> ()  [unwired: 1 in, 3 out]
      }
      frame "Clear Memory" {
        w229 = waveform(dbl)[] [] ("History Data")
        n86 = property on="Overview Chart" class="WFChart (strict)"("History Data"=waveform(dbl)[][] []) -> ()  [unwired: 2 in, 2 out]
        n87 = Enqueue Element(queue=w228, element=Data_Producer_States."Default", error in (no error)=w227) -> ()  [unwired: 1 in, 3 out]
        n88 = property on="Channel 0 Chart" class="WFChart (strict)"("History Data"=w229) -> ()  [unwired: 2 in, 2 out]
        n89 = property on="Channel 1 Chart" class="WFChart (strict)"("History Data"=w229) -> ()  [unwired: 2 in, 2 out]
        n90 = property on="Channel 3 Chart" class="WFChart (strict)"("History Data"=w229) -> ()  [unwired: 2 in, 2 out]
        n91 = property on="Channel 2 Chart" class="WFChart (strict)"("History Data"=w229) -> ()  [unwired: 2 in, 2 out]
      }
      frame "Exit" {
        n92 = Enqueue Element(queue=w239, element=Data_Producer_States."Exit", error in (no error)=w238) -> ()  [unwired: 1 in, 3 out]
      }
      frame "Default", Default {
        n93 = Enqueue Element(queue=w247, element=Data_Producer_States."Default", error in (no error)=w246) -> ()  [unwired: 1 in, 3 out]
      }
      frame "Create File" {
        w253 = T8."Disabled and Grayed Out" ("Disabled")
        # "Channel 3"
        # "Channel 2"
        # "Channel 1"
        # "Channel 0"
        n94 = Enqueue Element(queue=w260, element=Data_Producer_States."Read Data", error in (no error)=w259) -> ()  [unwired: 1 in, 3 out]
        n95 = Unbundle(w278) -> ("Use Channel 0"=w271:bool, "Use Channel 1"=w270:bool, "Use Channel 2"=w269:bool, "Use Channel 3"=w268:bool)
        n96 = call "File Creator.vi"("prompt"="Create a File for Channel 0", "Amplifier Channel 1"="Amplifier Channel 0", "User Data Channel 1"="User Data Channel 0", "Use Channel in"=w271) -> ("Refnum out"=w267:refnum<k34>)  [unwired: 7 in]
        n97 = call "File Creator.vi"("prompt"="Create a File for Channel 1", "Amplifier Channel 1"="Amplifier Channel 1", "User Data Channel 1"="User Data Channel 1", "Use Channel in"=w270) -> ("Refnum out"=w266:refnum<k34>)  [unwired: 7 in]
        n98 = call "File Creator.vi"("Amplifier Channel 1"="Amplifier Channel 2", "User Data Channel 1"="User Data Channel 2", "Use Channel in"=w269) -> ("Refnum out"=w265:refnum<k34>)  [unwired: 8 in]
        n99 = call "File Creator.vi"("Amplifier Channel 1"="Amplifier Channel 3", "User Data Channel 1"="User Data Channel 3", "Use Channel in"=w268) -> ("Refnum out"=w264:refnum<k34>)  [unwired: 8 in]
        n100 = Bundle("Refnum out"=w267, "Refnum out"=w266, "Refnum out"=w265, "Refnum out"=w264) -> (w261:T10)  [unwired: 1 in]
        n101 = Get Date/Time String(date format (0)=enum16{"short", "long", "abbreviated"}."short") -> (date string=→"Date mm/dd/yy":string, time string=→"Start Time hr/min":string)  [unwired: 2 in]
        n102 = property on="Preview Button" class="Bool (strict)"("DisabledEnum"=w253) -> ()  [unwired: 2 in, 2 out]
        n103 = property on="Clear Display" class="Bool"("DisabledEnum"=w253) -> ()  [unwired: 2 in, 2 out]
      }
      frame "End File" {
        w287 = T8."Enabled" ("Disabled")
        n104 = call "Functional Global I32.vi"("Enum"=enum16{"Set Data", "Get Data"}."Get Data") -> ("Integer"=w285:i32)  [unwired: 10 in]
        n105 = call "File Footer Writer.vi"("Old Data"=w298, "TDMS File Cluster"=w299, "Sample Rate"=w285, "In Use Cluster"=w300) -> ()  [unwired: 8 in]
        n106 = Enqueue Element(queue=w293, element=Data_Producer_States."Default", error in (no error)=w292) -> ()  [unwired: 1 in, 3 out]
        n107 = property on="Clear Display" class="Bool"("DisabledEnum"=w287) -> ()  [unwired: 2 in, 2 out]
        n108 = property on="Preview Button" class="Bool (strict)"("DisabledEnum"=w287) -> ()  [unwired: 2 in, 2 out]
        n109 = One Button Dialog(message="Recording is Finished") -> ()  [unwired: 1 in, 1 out]
      }
      frame "Preview" {
        w307 = u8 0 ("X Scale.Scale Fit")
        n110 = Dequeue Element(queue=w328, error in (no error)=w327) -> (element=w326:dbl[][])  [unwired: 1 in, 3 out]
        n111 = call "Functional Global I32.vi"("Enum"=enum16{"Set Data", "Get Data"}."Get Data") -> ("Integer"=w305:i32)  [unwired: 10 in]
        n112 = Enqueue Element(queue=w312, element=Data_Producer_States."Read Data", error in (no error)=w311) -> ()  [unwired: 1 in, 3 out]
        n113 = Reciprocal(x=w305) -> (1/x=w324:dbl)
        n114 = Index Array(array=w320, index (row)=0) -> (element=w318:dbl[])  [unwired: 1 in]
        n115 = Array Size(array=w318) -> (size(s)=w317:i32)
        n116 = property on="Recording Time (s)" class="DigNum (strict)"() -> ("Value"=w304:dbl)  [unwired: 2 in, 2 out]
        n117 = Multiply(x=20.0, y=w324) -> (x*y=w321:dbl)
        n118 = Multiply(x=w304, y=w305) -> (x*y=w303:dbl)
        n119 = To Quad Integer(1:w303) -> (0:w302:i64)
        n120 = Multiply(x=w317, y=w321) -> (x*y=w316:dbl)
        n121 = call "Preview Waveforms.vi"("Max Size"=w302, "Change in Time"=w321, "In Use Cluster"=w325, "Input Read Data"=w326, "Input Decimated Data"=w320) -> ("Output Waveform Cluster"=w306:T13, "Output Data"=w322:dbl[][])  [unwired: 5 in]
        n122 = Less?(x=w316, y=w304) -> (x < y?=w315:bool)
        n123 = property on="Overview Chart" class="WFChart (strict)"("XScale.ScaleFit"=w307) -> ()  [unwired: 2 in, 2 out]
        n124 = property on="Channel 0 Chart" class="WFChart (strict)"("XScale.ScaleFit"=w307) -> ()  [unwired: 2 in, 2 out]
        n125 = property on="Channel 1 Chart" class="WFChart (strict)"("XScale.ScaleFit"=w307) -> ()  [unwired: 2 in, 2 out]
        n126 = property on="Channel 2 Chart" class="WFChart (strict)"("XScale.ScaleFit"=w307) -> ()  [unwired: 2 in, 2 out]
        n127 = property on="Channel 3 Chart" class="WFChart (strict)"("XScale.ScaleFit"=w307) -> ()  [unwired: 2 in, 2 out]
        n128 = case shown="True" w315 {
          tunnel: [Consumer_Data__Consumer_Event_Com."Clear Memory" Consumer_Data__Consumer_Event_Com."Preview"] -> w314
          frame False {
          }
          frame True {
          }
        }
      }
    }
    n129 = Get Notifier Status(notifier=w150, error in (no error)=w149) -> (current notification=w148:bool)  [unwired: 4 out]
    n130 = Unbundle(w142) -> ("Waveform"=→"Channel 0 Chart":waveform(dbl), "Waveform"=→"Channel 1 Chart":waveform(dbl), "Waveform"=→"Channel 2 Chart":waveform(dbl), "Waveform"=→"Channel 3 Chart":waveform(dbl), →"Overview Chart":waveform(dbl)[])
    n131 = Or(x=w151, y=w148) -> (x .or. y?=w152:bool)
  }
  n132 = while {
    tunnel: w29 -> [w354]
    tunnel: w28 -> [w351]
    tunnel: [w353] -> w25
    tunnel: [w352] -> w24
    shift-right: [w339] -> _
    shift-left: Data_Producer_States."Default" -> [w332]
    shift-right: [w350] -> w18
    shift-left: _ -> [w348]
    shift-right: [w349] -> w17
    shift-left: _ -> [w347]
    tunnel: w10 -> [w344]
    tunnel: w9 -> [w343]
    shift-right: [w337] -> _
    shift-left: 0 -> [w338]
    tunnel: w3 -> [w334]
    tunnel: w2 -> [w333]
    stop <- w336 stop-if-true
    # "Producer Loop (Data)"
    n133 = Wait Until Next ms Multiple(millisecond multiple=u32 20) -> ()  [unwired: 1 out]
    n134 = Dequeue Element(queue=w344, timeout in ms (-1)=20, error in (no error)=w343) -> (element=w331:T2, timed out?=w342:bool)  [unwired: 2 out]
    n135 = Select(t=w332, s=w342, f=w331) -> (s? t:f=w341:T2)
    "Data Producer State" <- w341
    n136 = case shown="\"Read Data\"" w341 {
      tunnel: w354 -> [w368 w379 w389 w400]
      tunnel: [w366 w379 w389 w400] -> w353
      tunnel: [w365 w378 w388 w401] -> w352
      tunnel: w351 -> [w367 w378 w388 w401]
      tunnel: [w370 w377 w390 w402] -> w350
      tunnel: [w369 w376 w380 w403] -> w349
      tunnel: w348 -> [w372 w377 _ w402]
      tunnel: w347 -> [w371 w376 _ w403]
      tunnel: [FALSE FALSE FALSE TRUE] -> w345
      tunnel: [Data_Producer_States."Read Data" Data_Producer_States."Default" T15."Default" Data_Producer_States."Default"] -> w339
      tunnel: w338 -> [w361 _ _ _]
      tunnel: [w360 0 0 0] -> w337
      frame "Read Data" {
        n137 = call "Functional Global I32.vi"("Enum"=enum16{"Set Data", "Get Data"}."Get Data") -> ("Integer"=w357:i32)  [unwired: 10 in]
        n138 = Divide(x=w357, y=10) -> (x/y=w356:dbl)
        n139 = call-poly <vilib>:"DAQmxBase Read.vi"("task/channels in"=w372, "number of samples per channel"=w356, "timeout"=100.0, "error in"=w371) -> ("task out"=w370:refnum<k21>, "data"=w355:dbl[][], "error out"=w369:errorcluster)  [unwired: 9 in]
        n140 = Increment(x=w361) -> (x+1=w360:i32)
        "Read Data" <- w360
        n141 = Enqueue Element(queue=w368, element=w355, error in (no error)=w367) -> (queue out=w366:refnum<queue>, error out=w365:errorcluster)  [unwired: 1 in, 1 out]
      }
      frame "Default", Default {
      }
      frame "Set Sample Clock" {
        w381 = 10123 items=["Finite Samples"=10178, "Continuous Samples"=10123, "Hardware Timed Single Point"=12522] ("sample mode")
        n142 = property on="Sample Rate" class="DigNum (strict)"("DisabledEnum"=T8."Disabled and Grayed Out" ("Disabled")) -> ()  [unwired: 2 in, 2 out]
        n143 = call <vilib>:"DAQmxBase Create Task.vi"() -> ("task out"=w396:refnum<k21>, "error out"=w395:errorcluster)  [unwired: 14 in]
        n144 = call-poly <vilib>:"DAQmxBase Create Virtual Channel.vi"("task in"=w396, "physical channels"=tag "Dev1/ai0,Dev1/ai1,Dev1/ai2,Dev1/ai3", "error in"=w395) -> ("task out"=w393:refnum<k21>, "error out"=w394:errorcluster)  [unwired: 11 in]
        n145 = call-poly <vilib>:"DAQmxBase Timing.vi"("task/channels in"=w393, "sample mode"=w381, "rate"="Sample Rate", "error in"=w394) -> ("task out"=w392:refnum<k21>, "error out"=w391:errorcluster)  [unwired: 10 in]
        n146 = call "Functional Global I32.vi"("Enum"=enum16{"Set Data", "Get Data"}."Set Data", "Integer In"="Sample Rate") -> ()  [unwired: 9 in, 1 out]
        n147 = call <vilib>:"DAQmxBase Start Task.vi"("task/channels in"=w392, "error in"=w391) -> ("task out"=w390:refnum<k21>, "error out"=w380:errorcluster)  [unwired: 12 in]
        n148 = call <vilib>:"Simple Error Handler.vi"("error in (no error)"=w380) -> ()  [unwired: 4 in, 5 out]
      }
      frame "Exit" {
      }
    }
    n149 = Get Notifier Status(notifier=w334, error in (no error)=w333) -> (current notification=w335:bool)  [unwired: 4 out]
    n150 = Or(x=w345, y=w335) -> (x .or. y?=w336:bool)
  }
  n151 = Release Queue(queue=w27, error in (no error)=w26) -> ()  [unwired: 1 in, 3 out]
  n152 = Release Queue(queue=w25, error in (no error)=w24) -> (error out=w16:errorcluster)  [unwired: 1 in, 2 out]
  n153 = call <vilib>:"DAQmxBase Clear Task.vi"("task in"=w18, "error in"=w17) -> ("error out"=w15:errorcluster)  [unwired: 13 in]
  n154 = Merge Errors(w16, w15) -> (w14:errorcluster)
  n155 = call <vilib>:"Simple Error Handler.vi"("error in (no error)"=w14) -> ()  [unwired: 4 in, 5 out]
